vi "Michelle Prime (10-2).vi"() -> ()   [LabVIEW 2012]
panel:
  out "Boolean":bool
  in  "Numeric":dbl
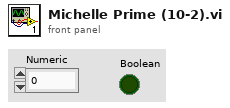
[diagram p1: front panel]
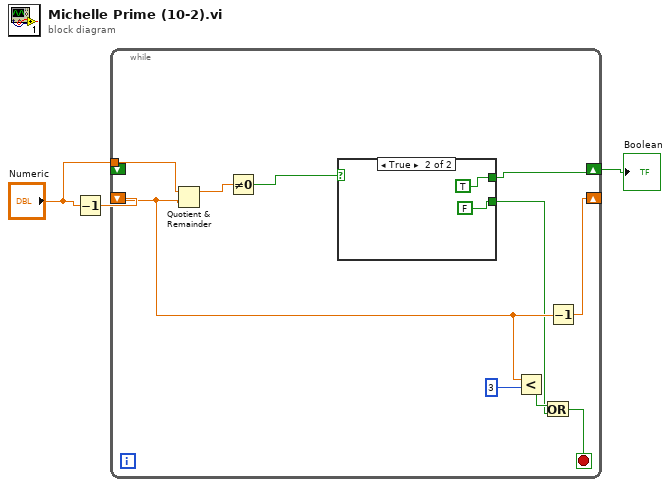
[diagram p0: block diagram]
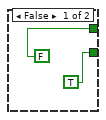
[diagram p2: hidden frame]
diagram:
  n1 = Decrement(x="Numeric") -> (x-1=w3:dbl)
  n2 = while {
    shift-right: [w13] -> _
    shift-left: w3 -> [w8]
    tunnel: "Numeric" -> [w11]
    shift-right: [w4] -> w1
    shift-left: _ -> [_]
    stop <- w7 stop-if-true
    n3 = Quotient & Remainder(x=w11, y=w8) -> (x-y*floor(x/y)=w12:dbl)  [unwired: 1 out]
    n4 = Not Equal To 0?(x=w12) -> (x != 0?=w10:bool)
    n5 = case shown="True" w10 {
      tunnel: [TRUE FALSE] -> w5
      tunnel: [FALSE TRUE] -> w4
      frame False {
      }
      frame True {
      }
    }
    n6 = Less?(x=w8, y=3) -> (x < y?=w6:bool)
    n7 = Or(x=w6, y=w5) -> (x .or. y?=w7:bool)
    n8 = Decrement(x=w8) -> (x-1=w13:dbl)
  }
  "Boolean" <- w1
